vi "LPF_2_ZPK.vi"(8 "error in (no error)":errorcluster, 11 "LPF params":T2) -> (0 "error out":errorcluster, 3 "ZPK model":T1)   [LabVIEW 2020, in "PC-RT_Controller.lvlib"]
doc: "Convert low pass filter parameters (f_Lpf [Hz], zeta) into continuous time zero-pole-gain (ZPK) model."
uses:
  PC-RT_Controller.lvlib
  TypeDefs/LPF params.ctl
  TypeDefs/ZPK_model.ctl
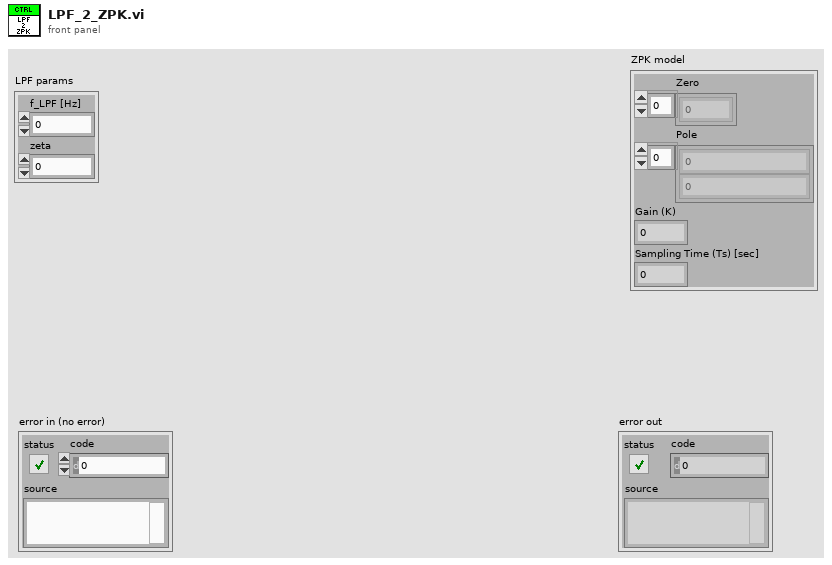
[diagram p1: front panel]
types:
  T1 = typedef "PC-RT_Controller.lvlib/ZPK_model.ctl" = cluster{"Zero":cdb[], "Pole":cdb[], "Gain (K)":dbl, "Sampling Time (Ts) [sec]":dbl}
  T2 = typedef "PC-RT_Controller.lvlib/LPF params.ctl" = cluster{"f_LPF [Hz]":dbl, "zeta":dbl}
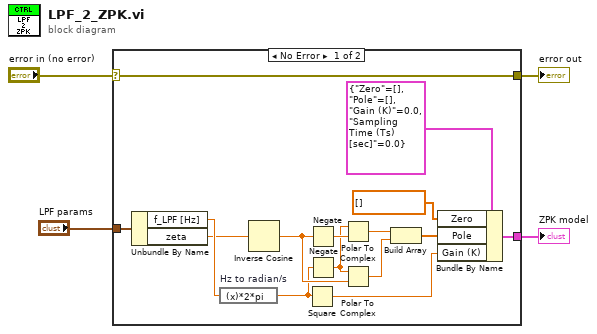
[diagram p0: block diagram]
diagram:
  n1 = case shown="No Error" "error in (no error)" {
    selector: "error in (no error)" -> [w8 w20]
    tunnel: [w10 _] -> w4
    tunnel: "LPF params" -> [w9 _]
    tunnel: [w8 w20] -> w1
    frame No Error {
      n2 = Unbundle By Name(w9) -> ("f_LPF [Hz]"=w19:dbl, "zeta"=w18:dbl)
      n3 = expression code="(x)*2*pi" "Hz to radian/s"(w19) -> (w5:dbl)
      n4 = Inverse Cosine(1:w18) -> (0:w16:dbl)
      n5 = Square(x=w5) -> (x^2=w11:dbl)
      n6 = Negate(x=w16) -> (-x=w15:dbl)
      n7 = Negate(x=w5) -> (-x=w6:dbl)
      n8 = Polar To Complex(1:w15, 2:w6) -> (0:w13:cdb)
      n9 = Polar To Complex(1:w16, 2:w6) -> (0:w14:cdb)
      n10 = Build Array(w13, w14) -> (w12:cdb[])
      n11 = Bundle By Name(cluster=T1 {"Zero"=[], "Pole"=[], "Gain (K)"=0.0, "Sampling Time (Ts) [sec]"=0.0} ("ZPK model"), "Zero"=cdb[] [], "Pole"=w12, "Gain (K)"=w11) -> (w10:T1)
    }
    frame Error {
    }
  }
  "ZPK model" <- w4
  "error out" <- w1
